vi "DUAL GAUGE-Parameter Control.vi"(7 "W/R":bool, 8 "Fehler (Eingang)":errorcluster, 9 "Parameter Save":i8(ring)=2 items=["User", "default", "no change"], 10 "Parameter lock":i8(ring)=2 items=["Off", "On", "no change"], 11 "Referenz in":refnum<visa-resource-name>) -> (0 "Cluster (Ausgang)":errorcluster, 2 "Parameter lock Get":i8(ring) items=["Off", "On"], 3 "Referenz out":refnum<visa-resource-name>)   [LabVIEW 2013, in "Dual Gauge.lvlib"]
uses:
  Dual Gauge.lvlib
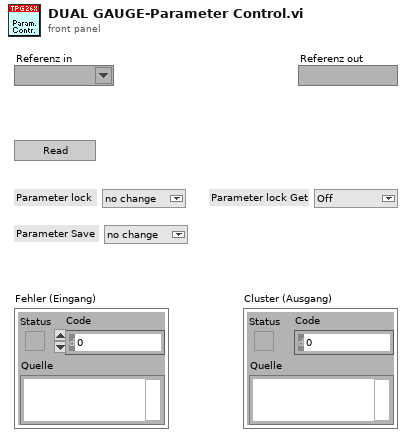
[diagram p1: front panel]
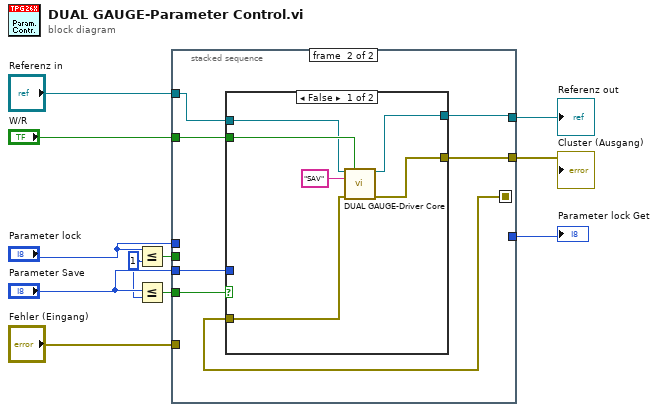
[diagram p0: block diagram]
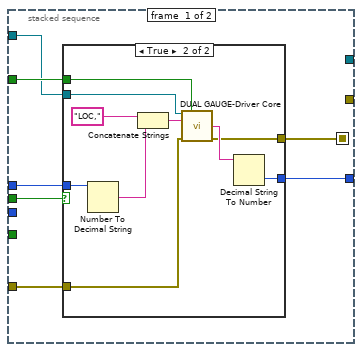
[diagram p2: hidden frame]
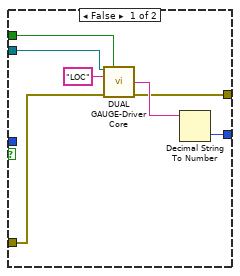
[diagram p3: hidden frame]
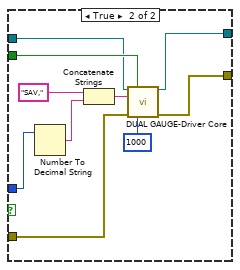
[diagram p4: hidden frame]
diagram:
  w7 = i8 1 ("y")
  n1 = Less Or Equal?(x="Parameter lock", y=w7) -> (x <= y?=w6:bool)
  n2 = Less Or Equal?(x="Parameter Save", y=w7) -> (x <= y?=w5:bool)
  n3 = stacked-sequence {
    seq-local: [w12 _] -> [_ w39]
    tunnel: "W/R" -> [w18 w42]
    tunnel: [w17 _] -> w8
    tunnel: "Parameter lock" -> [w16 _]
    tunnel: w5 -> [_ w41]
    tunnel: "Parameter Save" -> [_ w40]
    tunnel: w6 -> [w15 _]
    tunnel: "Referenz in" -> [w14 w38]
    tunnel: "Fehler (Eingang)" -> [w13 _]
    tunnel: [_ w37] -> w2
    tunnel: [_ w36] -> w1
    frame #0 {
      n4 = case shown="True" w15 {
        tunnel: w18 -> [w24 w34]
        tunnel: [w23 w31] -> w17
        tunnel: w16 -> [_ w30]
        tunnel: [w22 w29] -> w12
        tunnel: w14 -> [w20 w27]
        tunnel: w13 -> [w19 w26]
        frame False {
          n5 = call "DUAL GAUGE-Driver Core.vi"("Referenz in"=w20, "Write/Read"=w24, "Command"="LOC", "Fehler (Eingang)"=w19) -> ("String Out"=w25:string, "Cluster (Ausgang)"=w22:errorcluster)  [unwired: 9 in, 1 out]
          n6 = Decimal String To Number(string=w25) -> (number=w23:i32)  [unwired: 2 in, 1 out]
        }
        frame True {
          n7 = Number To Decimal String(number=w30) -> (decimal integer string=w33:string)  [unwired: 1 in]
          n8 = Concatenate Strings("LOC,", w33) -> (w28:string)
          n9 = call "DUAL GAUGE-Driver Core.vi"("Referenz in"=w27, "Write/Read"=w34, "Command"=w28, "Fehler (Eingang)"=w26) -> ("String Out"=w35:string, "Cluster (Ausgang)"=w29:errorcluster)  [unwired: 9 in, 1 out]
          n10 = Decimal String To Number(string=w35) -> (number=w31:i32)  [unwired: 2 in, 1 out]
        }
      }
    }
    frame #1 {
      n11 = case shown="False" w41 {
        tunnel: w42 -> [w48 w58]
        tunnel: w40 -> [_ w55]
        tunnel: [w47 w54] -> w36
        tunnel: w39 -> [w45 w51]
        tunnel: w38 -> [w44 w50]
        tunnel: [w43 w49] -> w37
        frame False {
          n12 = call "DUAL GAUGE-Driver Core.vi"("Referenz in"=w44, "Write/Read"=w48, "Command"="SAV", "Fehler (Eingang)"=w45) -> ("Referenz out"=w43:refnum<visa-resource-name>, "Cluster (Ausgang)"=w47:errorcluster)  [unwired: 9 in, 1 out]
        }
        frame True {
          n13 = Number To Decimal String(number=w55) -> (decimal integer string=w57:string)  [unwired: 1 in]
          n14 = Concatenate Strings("SAV,", w57) -> (w52:string)
          n15 = call "DUAL GAUGE-Driver Core.vi"("Referenz in"=w50, "Write/Read"=w58, "Command"=w52, "Fehler (Eingang)"=w51, "Timeout [ms]"=u32 1000) -> ("Referenz out"=w49:refnum<visa-resource-name>, "Cluster (Ausgang)"=w54:errorcluster)  [unwired: 8 in, 1 out]
        }
      }
    }
  }
  "Parameter lock Get" <- w8
  "Referenz out" <- w2
  "Cluster (Ausgang)" <- w1
